vi "SynchroResolver Simulation Velocity.vi"() -> ()   [LabVIEW 8.6]
uses:
  vi.lib/UeiDaq/UeiDaqReadOneScaledScan.vi
  <libdir>/resource/objmgr/ueidaq.rc
  vi.lib/UeiDaq/UeiDaqConfigureTimingForSimpleIO.vi
  vi.lib/UeiDaq/UeiDaqCreateSimulatedSynchroResolverSession.vi
  vi.lib/UeiDaq/UeiDaqCreateSynchroResolverSession.vi
panel:
  out "Delay (us)":dbl
  in  "Number of revolutions":i32
  out "Available":i32[](array[numeric])
  out "Written":i32[](array[numeric])
  in  "Number of steps per rev.":i32
  in  "Velocity (RPM)":dbl
  in  "Mode":enum16{"Synchro", "Resolver"}(ring)
  out "Measured Excitation Frequency":dbl[](array[numeric])
  out "Measured Excitation Amplitude":dbl[](array[numeric])
  in  "Excitation frequency":dbl
  in  "Excitation amplitude":dbl
  in  "Simulated Output Resource":string
  out "Measured Synchro/Resolver position":dbl[][](graph)
  in  "Refresh rate (ms)":u32
  in  "stop":bool
  in  "Input Resource":string
  # "Synchro/Resolver Simulation"
  # "This example takes advantage of the Synchro/Resolver simulation capability on the AI-255.It Simulates a Synchro or a Resolver out of channel 1 and measures it back on channel 0. You need to connect the folowing pins:\nCh0 IN A- <--> Ch1 OUT A-\nCh0 IN A+ <--> Ch1 OUT A+\nCh0 IN B- <--> Ch1 OUT B-\nCh0 IN B+ <--> Ch1 OUT B+\nCh0 IN C- <--> Ch1 OUT C-\nCh0 IN C+ <--> Ch1 OUT C+\nCh0 OUT D- <--> Ch1 IN D-\nCh0 OUT D+ <--> Ch1 IN D+"
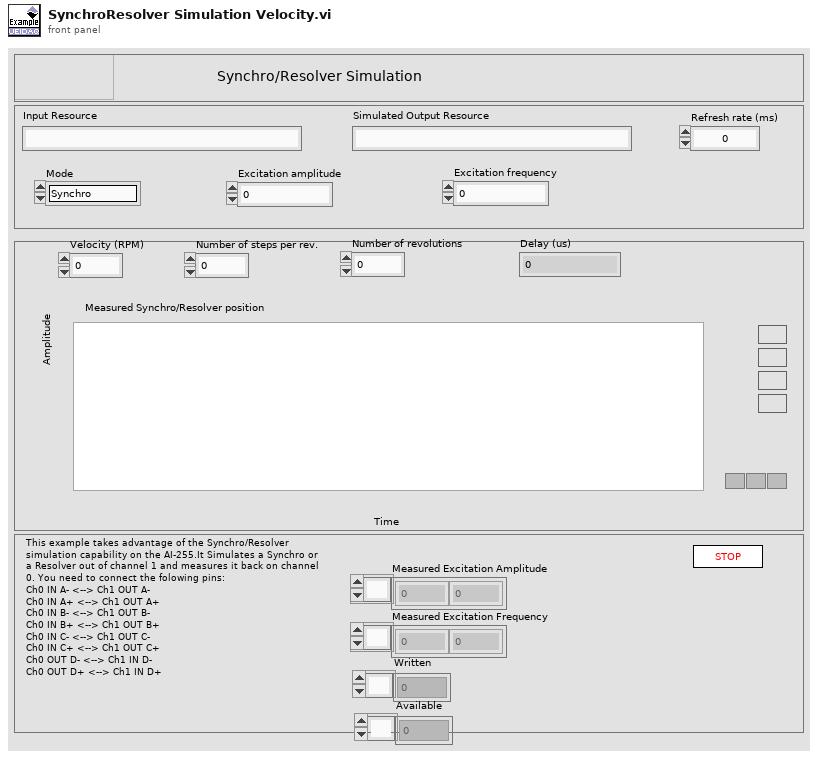
[diagram p1: front panel]
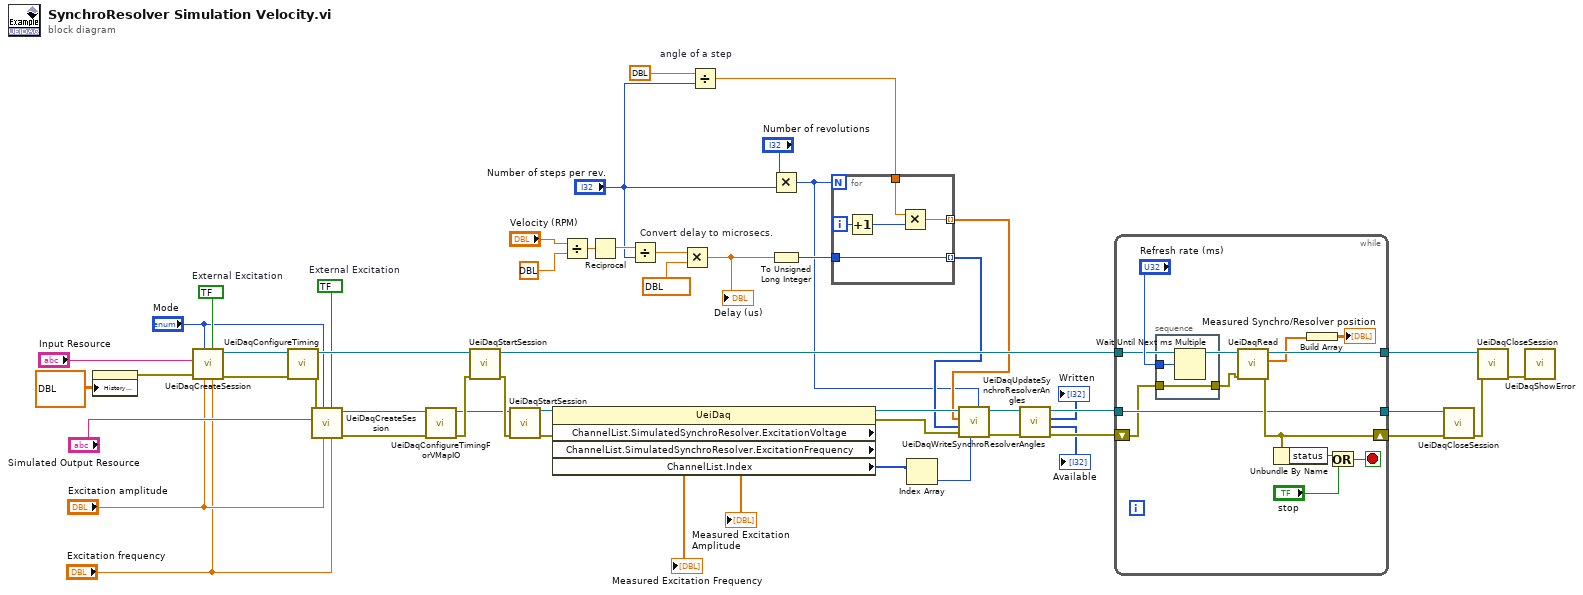
[diagram p0: block diagram]
diagram:
  w26 = bool ?  # External Excitation
  w28 = bool ?  # External Excitation
  n1 = property on="Measured Synchro/Resolver position" class="WFChart (strict)"("History Data"=dbl[][] ?) -> (error out=w41:errorcluster)  [unwired: 2 in, 1 out]
  n2 = call-poly "UeiDaqCreateSession.vi"("Excitation frequency"="Excitation frequency", "External Excitation"=w28, "Excitation voltage"="Excitation amplitude", "Mode"="Mode", "error in (no error)"=w41, "Resource"="Input Resource") -> ("error out"=w49:errorcluster, "UeiDaq Refnum Out"=w47:refnum<k20>)  [unwired: 1 in, 3 out]
  n3 = call-poly "UeiDaqConfigureTiming.vi"("error in (no error)"=w49, "UeiDaq Refnum In"=w47) -> ("error out"=w40:errorcluster, "UeiDaq Refnum Out"=w39:refnum<k20>)  [unwired: 8 out]
  n4 = call-poly "UeiDaqCreateSession.vi"("Excitation frequency"="Excitation frequency", "External Excitation"=w26, "Excitation voltage"="Excitation amplitude", "Mode"="Mode", "error in (no error)"=w40, "Resource"="Simulated Output Resource") -> ("error out"=w51:errorcluster, "UeiDaq Refnum Out"=w52:refnum<k20>)  [unwired: 1 in, 3 out]
  n5 = call "UeiDaqConfigureTimingForVMapIO.vi"("error in (no error)"=w51, "UeiDaq Refnum In"=w52) -> ("error out"=w37:errorcluster, "UeiDaq Refnum Out"=w35:refnum<k20>)  [unwired: 8 in]
  n6 = call "UeiDaqStartSession.vi"("error in (no error)"=w37, "UeiDaq Refnum In"=w39) -> ("error out"=w36:errorcluster, "UeiDaq Refnum Out"=w38:refnum<k20>)  [unwired: 8 out]
  n7 = call "UeiDaqStartSession.vi"("error in (no error)"=w36, "UeiDaq Refnum In"=w35) -> ("error out"=w33:errorcluster, "UeiDaq Refnum Out"=w34:refnum<k20>)  [unwired: 8 out]
  n8 = property class="UeiDaq"(reference=w34, error in=w33) -> (reference out=w25:refnum<k20>, error out=w20:errorcluster, "ChannelList.SimulatedSynchroResolver.ExcitationVoltage"=→"Measured Excitation Amplitude":dbl[], "ChannelList.SimulatedSynchroResolver.ExcitationFrequency"=→"Measured Excitation Frequency":dbl[], "ChannelList.Index"=w12:i32[])
  n9 = Divide(x="Velocity (RPM)", y=dbl ?) -> (x/y=w15:dbl)
  n10 = Reciprocal(x=w15) -> (1/x=w14:dbl)
  n11 = Divide(x=w14, y="Number of steps per rev.") -> (x/y=w5:dbl)
  n12 = Multiply "Convert delay to microsecs."(x=w5, y=dbl ?) -> (x*y=w7:dbl)
  "Delay (us)" <- w7
  n13 = Divide "angle of a step"(x=dbl ?, y="Number of steps per rev.") -> (x/y=w18:dbl)
  n14 = Multiply(x="Number of revolutions", y="Number of steps per rev.") -> (x*y=w1:i32)
  n15 = To Unsigned Long Integer(number=w7) -> (unsigned 32bit integer=w4:u32)
  n16 = for {
    N: w1 -> [_]
    tunnel: w18 -> [w58]
    tunnel: [w57] -> w13 mode=indexing
    tunnel: w4 -> [w56]
    tunnel: [w56] -> w3 mode=indexing
    i -> [w55]
    n17 = Increment(x=w55) -> (x+1=w54:i32)
    n18 = Multiply(x=w58, y=w54) -> (x*y=w57:dbl)
  }
  n19 = Index Array(array=w12) -> (element=w11:i32)  [unwired: 1 in]
  n20 = call "UeiDaqWriteSynchroResolverAngles.vi"("Number of values"=w1, "Channel"=w11, "error in (no error)"=w20, "Delays (us)"=w3, "Angles (rad)"=w13, "UeiDaq Refnum In"=w25) -> ("error out"=w24:errorcluster, "UeiDaq Refnum Out"=w22:refnum<k20>)  [unwired: 4 in]
  n21 = call "UeiDaqUpdateSynchroResolverAngles.vi"("error in (no error)"=w24, "UeiDaq Refnum In"=w22) -> ("error out"=w23:errorcluster, "Available"=→"Available":i32[], "Written"=→"Written":i32[], "UeiDaq Refnum Out"=w21:refnum<k20>)  [unwired: 6 in]
  n22 = while {
    tunnel: w21 -> [w61]
    tunnel: [w61] -> w53
    tunnel: w38 -> [w65]
    tunnel: [w67] -> w46
    shift-right: [w63] -> w45
    shift-left: w23 -> [w60]
    stop <- w69 stop-if-true
    n23 = stacked-sequence {
      tunnel: "Refresh rate (ms)" -> [w72]
      tunnel: w60 -> [w71]
      tunnel: [w71] -> w59
      frame #0 {
        n24 = Wait Until Next ms Multiple(millisecond multiple=w72) -> ()  [unwired: 1 out]
      }
    }
    n25 = call-poly "UeiDaqRead.vi"("error in (no error)"=w59, "UeiDaq Refnum In"=w65) -> ("error out"=w63:errorcluster, "Scaled Data"=w62:dbl[], "UeiDaq Refnum Out"=w67:refnum<k20>)  [unwired: 7 out]
    n26 = Unbundle By Name(w63) -> ("status"=w66:bool)
    n27 = Build Array(w62) -> (→"Measured Synchro/Resolver position":dbl[][])
    n28 = Or(x=w66, y="stop") -> (x .or. y?=w69:bool)
  }
  n29 = call "UeiDaqCloseSession.vi"("error in (no error)"=w45, "UeiDaq Refnum In"=w53) -> ("error out"=w44:errorcluster)  [unwired: 1 in, 8 out]
  n30 = call "UeiDaqCloseSession.vi"("error in (no error)"=w44, "UeiDaq Refnum In"=w46) -> ("error out"=w43:errorcluster)  [unwired: 1 in, 8 out]
  n31 = call "UeiDaqShowError.vi"("error in (no error)"=w43) -> ()  [unwired: 2 in, 9 out]
